vi "Auton Strafe.vi"(0 "Distance":dbl=3.0 format="%#_13g", 1 "PID gains":T1 {"derivative time (Td, min)" format="%.3f"; "integral time (Ti, min)" format="%.3f"; "proportional gain (Kc)" format="%.3f"}, 2 "PID Complete Delay":u32, 3 "Refnum in":refnum<k33>) -> (7 "Distance Travelled":dbl, 10 "rt fifo out":refnum<k33>)   [LabVIEW 2014]
uses:
  TeleopCmd.ctl
  CmdFlag.ctl
  AutonCals.vi
  encoderData.vi
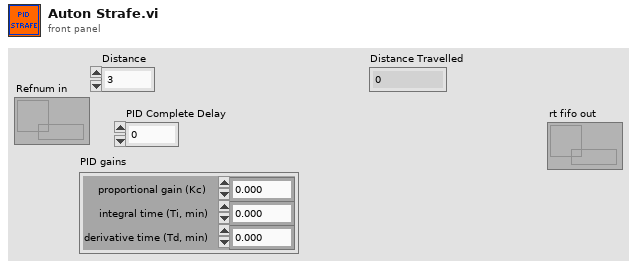
[diagram p1: front panel]
types:
  T1 = cluster{"proportional gain (Kc)":dbl, "integral time (Ti, min)":dbl, "derivative time (Td, min)":dbl}
  T2 = typedef "TeleopCmd.ctl" = cluster{"CmdFlag":T3, "throttle":dbl, "turn":dbl, "Override":bool, "Strafe":dbl, "MotorPwrMax":u8, "Time":u32, "ultrasonic override":bool}
  T3 = typedef "CmdFlag.ctl" = enum16{"noop", "logflag", "suspend", "resume"}
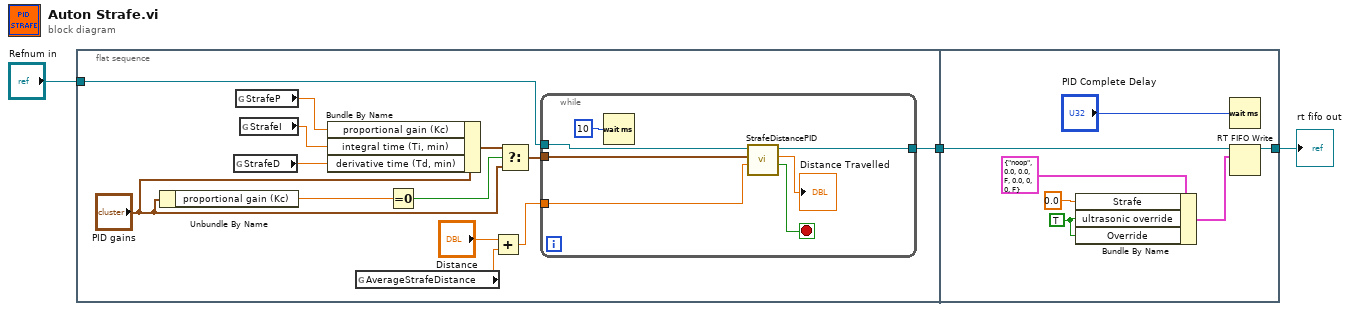
[diagram p0: block diagram]
diagram:
  n1 = flat-sequence {
    tunnel: "Refnum in" -> [w16]
    tunnel: [w7] -> w2
    tunnel: w2 -> [w27]
    tunnel: [w24] -> w1
    frame #0 {
      n2 = Unbundle By Name("PID gains") -> ("proportional gain (Kc)"=w11:dbl)
      n3 = global read "AutonCals.vi" "StrafeD"() -> (w14:dbl)
      n4 = global read "AutonCals.vi" "StrafeP"() -> (w13:dbl)
      n5 = global read "AutonCals.vi" "StrafeI"() -> (w15:dbl)
      n6 = Bundle By Name(cluster="PID gains", "proportional gain (Kc)"=w13, "integral time (Ti, min)"=w15, "derivative time (Td, min)"=w14) -> (w10:T1)
      n7 = global read "encoderData.vi" "AverageStrafeDistance"() -> (w6:dbl)
      n8 = Equal To 0?(x=w11) -> (x = 0?=w12:bool)
      n9 = Add(x="Distance", y=w6) -> (x+y=w4:dbl)
      n10 = Select(t=w10, s=w12, f="PID gains") -> (s? t:f=w8:T1)
      n11 = while {
        tunnel: w16 -> [w22]
        tunnel: w8 -> [w20]
        tunnel: [w19] -> w7
        tunnel: w4 -> [w17]
        stop <- w23 stop-if-true
        n12 = Wait (ms)(milliseconds to wait=u32 10) -> ()  [unwired: 1 out]
        n13 = call "StrafeDistancePID.vi"("Distance"=w17, "PID gains"=w20, "Refnum in"=w22) -> ("Boolean"=w23:bool, "Distance Travelled"=→"Distance Travelled":dbl, "Refnum out"=w19:refnum<k33>)  [unwired: 6 in]
      }
    }
    frame #1 {
      w28 = TRUE ("ultrasonic override")
      n14 = Bundle By Name(cluster=T2 {"CmdFlag"=enum."noop", "throttle"=0.0, "turn"=0.0, "Override"=FALSE, "Strafe"=0.0, "MotorPwrMax"=0, "Time"=0, "ultrasonic override"=FALSE} ("Cluster"), "Strafe"=0.0, "ultrasonic override"=w28, "Override"=w28) -> (w29:T2)
      n15 = Wait (ms)(milliseconds to wait="PID Complete Delay") -> ()  [unwired: 1 out]
      n16 = RT FIFO Write(0:w27, 1:w29) -> (8:w24:refnum<k33>)  [unwired: 3 in, 3 out]
    }
  }
  "rt fifo out" <- w1
